vi "AutoDrive.vi"(9 "Heading":dbl, 10 "Drive Y":dbl, 11 "Drive X":dbl) -> (0 "Done?":bool)   [LabVIEW 2014]
uses:
  Drivetrain Code/Drivetrain Mode.ctl
  Drivetrain Code/Drivetrain Control.ctl
  Robot Global Data.vi
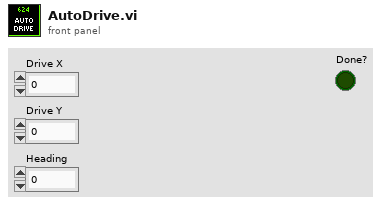
[diagram p1: front panel]
types:
  T1 = typedef "Drivetrain Control.ctl" = cluster{"Mode":T2, "X":dbl, "Y":dbl, "Heading Target":dbl, "Drive X":dbl, "Drive Y":dbl}
  T2 = typedef "Drivetrain Mode.ctl" = enum16{"Manual", "Gyro Steer", "Vision Steer", "Drive Distance"}
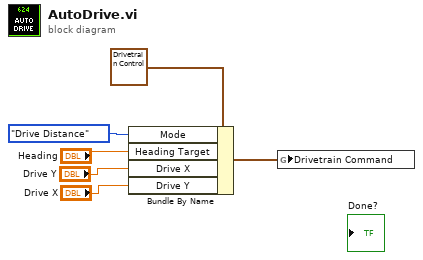
[diagram p0: block diagram]
diagram:
  n1 = Bundle By Name(cluster=T1 {"Mode"=enum."Gyro Steer", "X"=0.0, "Y"=0.0, "Heading Target"=0.0, "Drive X"=0.0, "Drive Y"=0.0} ("Drivetrain Command"), "Mode"=Drivetrain_Mode."Drive Distance", "Heading Target"="Heading", "Drive X"="Drive Y", "Drive Y"="Drive X") -> (w6:T1)
  n2 = global write "Robot Global Data.vi" "Drivetrain Command"(w6) -> ()
